vi "Bubble Sort Person Array Using Direct SubVI Call.vi"(11 "Unsorted":T1[](array[typedef]) {"Birth Date" format="%<%Y/%b/%d>T"}) -> (3 "Sorted":T1[](array[typedef]) {"Birth Date" format="%<%Y/%b/%d>T"})   [LabVIEW 2023]
doc: "This VI implements a basic Bubble Sort for the array data, using the provided VI reference as the comparison function for two elements."
uses:
  Person Information.ctl
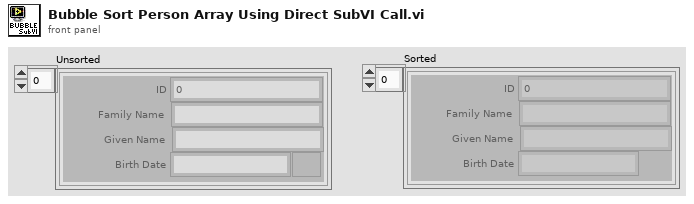
[diagram p1: front panel]
types:
  T1 = typedef "Person Information.ctl" = cluster{"ID":u32, "Family Name":string, "Given Name":string, "Birth Date":timestamp}
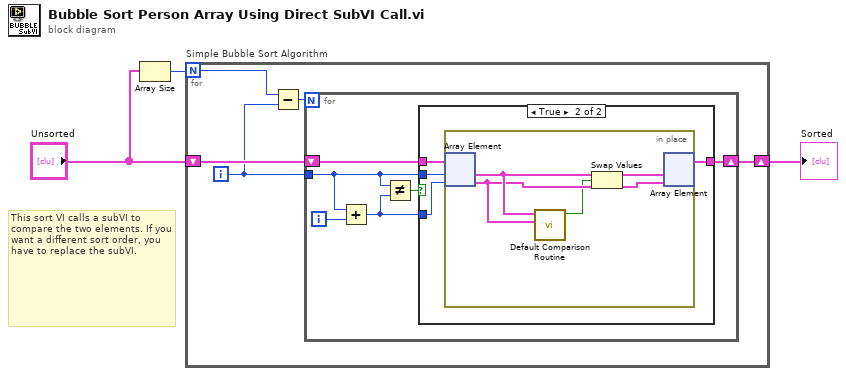
[diagram p0: block diagram]
diagram:
  # "This sort VI calls a subVI to compare the two elements. If you want a different sort order, you have to replace the subVI."
  n1 = Array Size(array="Unsorted") -> (size(s)=w3:i32)
  n2 = for "Simple Bubble Sort Algorithm" {
    N: w3 -> [w5]
    shift-right: [w7] -> w2
    shift-left: "Unsorted" -> [w8]
    i -> [w4]
    n3 = Subtract(x=w5, y=w4) -> (x-y=w6:i32)
    n4 = for {
      N: w6 -> [_]
      shift-right: [w13] -> w7
      shift-left: w8 -> [w14]
      tunnel: w4 -> [w9]
      i -> [w11]
      n5 = Add(x=w9, y=w11) -> (x+y=w10:i32)
      n6 = Not Equal?(x=w9, y=w10) -> (x != y?=w12:bool)
      n7 = case shown="True" w12 {
        tunnel: w14 -> [w15 w19]
        tunnel: [w15 w18] -> w13
        tunnel: w9 -> [_ w17]
        tunnel: w10 -> [_ w16]
        frame False {
        }
        frame True {
          n8 = in-place {
            n9 = in-place-array #1(w19, w17, w16) -> (w22:T1, w21:T1)
            n10 = call "Default Comparison Routine.vi"("Person B"=w21, "Person A"=w22) -> ("Swap?"=w20:bool)  [unwired: 9 in]
            n11 = Swap Values(12:w22, 13:w20, 14:w21) -> (1:w24:T1, 3:w23:T1)
            n12 = in-place-array #1(w24, w23) -> (w18:T1[])  [unwired: 2 out]
          }
        }
      }
    }
  }
  "Sorted" <- w2
